vi "get_objectData.vi"(0 "MoAgSy_Message.lvclass in":refnum<class "MoAgSy_Message.lvclass">, 5 "error in (no error)":errorcluster) -> (14 "MoAgSy_Message.lvclass out":refnum<class "MoAgSy_Message.lvclass">, 16 "Object Library":string, 17 "Object Class Name":string, 19 "error out":errorcluster)   [LabVIEW 2009, in "MoAgSy.lvlib" / "MoAgSy_Message.lvclass"]
uses:
  MoAgSy_Message.lvclass
  MoAgSy_Message.lvclass/MoAgSy_Message.ctl
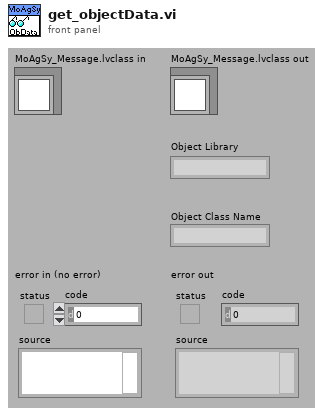
[diagram p1: front panel]
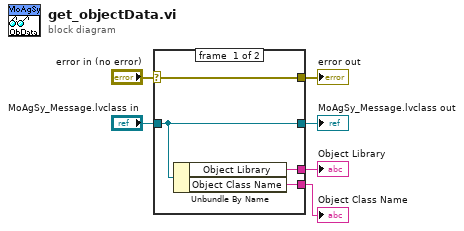
[diagram p0: block diagram]
diagram:
  n1 = case shown="No Error" "error in (no error)" {
    selector: "error in (no error)" -> [w10 w11]
    tunnel: [w10 w11] -> w5
    tunnel: [w9 w12] -> w3
    tunnel: "MoAgSy_Message.lvclass in" -> [w9 w12]
    tunnel: [w8 _] -> w2
    tunnel: [w7 _] -> w1
    frame #0 {
      n2 = Unbundle By Name(w9) -> ("Object Library"=w8:string, "Object Class Name"=w7:string)
    }
    frame #1 {
    }
  }
  "error out" <- w5
  "MoAgSy_Message.lvclass out" <- w3
  "Object Library" <- w2
  "Object Class Name" <- w1
